vi "Configure Measurement (Occupied Bandwidth).vi"(0 "VISA resource name":refnum<visa-resource-name>, 1 "Power Level (26 dB)":dbl=26.0, 5 "OBW Method (0: Percent)":i32(ring) items=["Percent", "dBc"], 9 "OBW Percent Power (99.00 %)":dbl=99.0, 11 "error in (no error)":errorcluster) -> (4 "VISA resource name out":refnum<visa-resource-name>, 15 "error out":errorcluster)   [LabVIEW 2022 SP3, in "Agilent N934X Series.lvlib"]
doc: "Sets the Occupied Bandwidth measurement parameters."
uses:
  <instrlib>/Agilent N934X Series/Agilent N934X Series.lvlib
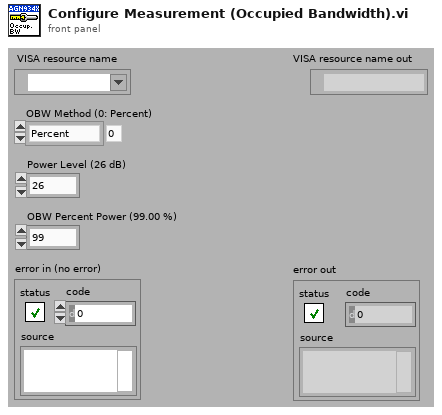
[diagram p1: front panel]
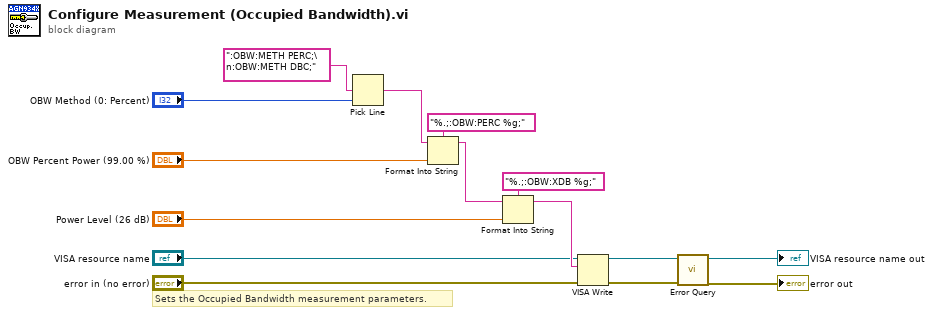
[diagram p0: block diagram]
diagram:
  # "Sets the Occupied Bandwidth measurement parameters."
  n1 = Pick Line(multi-line string=":OBW:METH PERC;\n:OBW:METH DBC;", line index="OBW Method (0: Percent)") -> (output string=w13:string)  [unwired: 1 in]
  n2 = Format Into String(format string="%.;:OBW:PERC %g;", initial string=w13, "OBW Percent Power (99.00 %)") -> (resulting string=w10:string)  [unwired: 1 in, 1 out]
  n3 = Format Into String(format string="%.;:OBW:XDB %g;", initial string=w10, "Power Level (26 dB)") -> (resulting string=w7:string)  [unwired: 1 in, 1 out]
  n4 = VISA Write(VISA resource name="VISA resource name", write buffer=w7, error in (no error)="error in (no error)") -> (VISA resource name out=w4:refnum<visa-resource-name>, error out=w3:errorcluster)  [unwired: 1 out]
  n5 = call <instrlib>:"Error Query.vi"("error in (no error)"=w3, "VISA resource name"=w4) -> ("error out"=→"error out":errorcluster, "VISA resource name out"=→"VISA resource name out":refnum<visa-resource-name>)  [unwired: 6 in, 2 out]
